vi "Get_Rois.vi"(8 "error in":errorcluster, 11 "camera handle in":u64) -> (0 "error out":errorcluster, 1 "rois":T1[](array[typedef]), 3 "camera handle out":u64)   [LabVIEW 2019, in "PICam.lvlib"]
doc: "Picam_SetParameterRoisValue() configures an Rois parameter to a specified value\nduring camera setup.\n\nIn this VI implementation we only want to specify a single ROI, so the input is a single ROI cluster!"
uses:
  PICam.lvlib
  Ctrls/PicamROI.ctl
  Picam64.dll
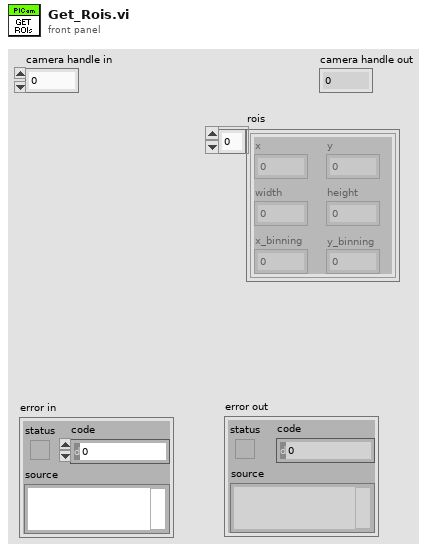
[diagram p1: front panel]
types:
  T1 = typedef "PICam.lvlib/PicamROI.ctl" = cluster{"x":i32, "width":i32, "x_binning":i32, "y":i32, "height":i32, "y_binning":i32}
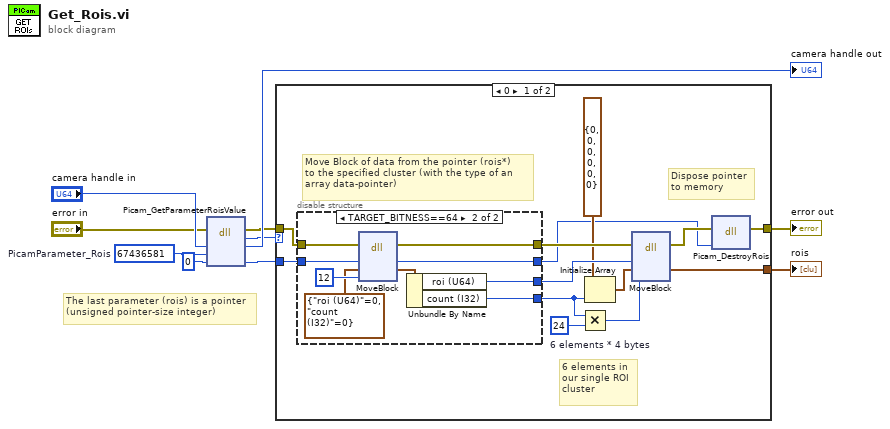
[diagram p0: block diagram]
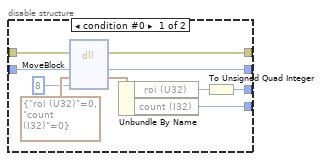
[diagram p2: hidden frame]
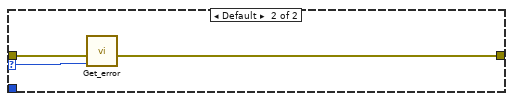
[diagram p3: hidden frame]
diagram:
  w8 = u32 67436581  # PicamParameter_Rois
  # "The last parameter (rois) is a pointer\n(unsigned pointer-size integer)"
  n1 = dll-call lib="Picam*.*" fn="Picam_GetParameterRoisValue"(error in="error in", "handle"="camera handle in", "param"=w8, "roid"=u64 0) -> (error out=w3:errorcluster, "return type"=w4:i32, "handle"=→"camera handle out":u64, "roid"=w2:u64)  [unwired: 3 in, 1 out]
  n2 = case shown="0" w4 {
    selector: w4 -> [_ w44]
    tunnel: [w12 w45] -> w10
    tunnel: w3 -> [w22 w43]
    tunnel: w2 -> [w23 _]
    tunnel: [w17 _] -> w1
    frame 0 {
      w16 = 24  # 6 elements * 4 bytes
      # "Move Block of data from the pointer (rois*)\nto the specified cluster (with the type of an\narray data-pointer)"
      # "Dispose pointer\nto memory"
      # "6 elements in\nour single ROI\ncluster"
      n3 = disable-structure shown="TARGET_BITNESS==64" {
        disable-tunnel: w23 -> [w33 w42]
        disable-tunnel: [w30 w40] -> w11
        disable-tunnel: w22 -> [w29 w39]
        disable-tunnel: [w28 w38] -> w21
        disable-tunnel: [w25 w35] -> w20
        disable-tunnel: [w24 w34] -> w15
        frame condition #0 {
          n4 = dll-call lib="LabVIEW" fn="MoveBlock"(error in=w29, "src"=w33, "dst"=cluster{"roi (U32)":u32, "count (I32)":i32} {"roi (U32)"=0, "count (I32)"=0}, "size"=u64 8 ("roid")) -> (error out=w28:errorcluster, "src"=w30:u64, "dst"=w27:cluster{"roi (U32)":u32, "count (I32)":i32})  [unwired: 4 in, 1 out]
          n5 = Unbundle By Name(w27) -> ("roi (U32)"=w26:u32, "count (I32)"=w24:i32)
          n6 = To Unsigned Quad Integer(1:w26) -> (0:w25:u64)
        }
        frame condition #1 (active) {
          n7 = dll-call lib="LabVIEW" fn="MoveBlock"(error in=w39, "src"=w42, "dst"=cluster{"roi (U64)":u64, "count (I32)":i32} {"roi (U64)"=0, "count (I32)"=0}, "size"=u64 12 ("roid")) -> (error out=w38:errorcluster, "src"=w40:u64, "dst"=w36:cluster{"roi (U64)":u64, "count (I32)":i32})  [unwired: 4 in, 1 out]
          n8 = Unbundle By Name(w36) -> ("roi (U64)"=w35:u64, "count (I32)"=w34:i32)
        }
      }
      n9 = Multiply(x=w15, y=w16) -> (x*y=w14:i32)
      n10 = Initialize Array(T1 {"x"=0, "width"=0, "x_binning"=0, "y"=0, "height"=0, "y_binning"=0} ("PicamROI"), w15) -> (w19:T1[])
      n11 = dll-call lib="LabVIEW" fn="MoveBlock"(error in=w21, "src"=w20, "dst"=w19, "size"=w14) -> (error out=w13:errorcluster, "dst"=w17:T1[])  [unwired: 5 in, 1 out]
      n12 = dll-call lib="Picam*.*" fn="Picam_DestroyRois"(error in=w13, "rois"=w11) -> (error out=w12:errorcluster)  [unwired: 4 in, 1 out]
    }
    frame Default {
      n13 = call "Get_error.vi"("PICam_Error"=w44, "error in (no error)"=w43) -> ("error out"=w45:errorcluster)  [unwired: 9 in]
    }
  }
  "error out" <- w10
  "rois" <- w1
